vi "find_path.vi"(11 "Array":i16[](array[numeric])) -> (0 "debug array":i32[](array[numeric]), 3 "Array 2":i32[](array[numeric]))   [LabVIEW 2012]
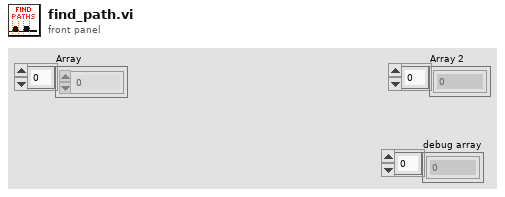
[diagram p1: front panel]
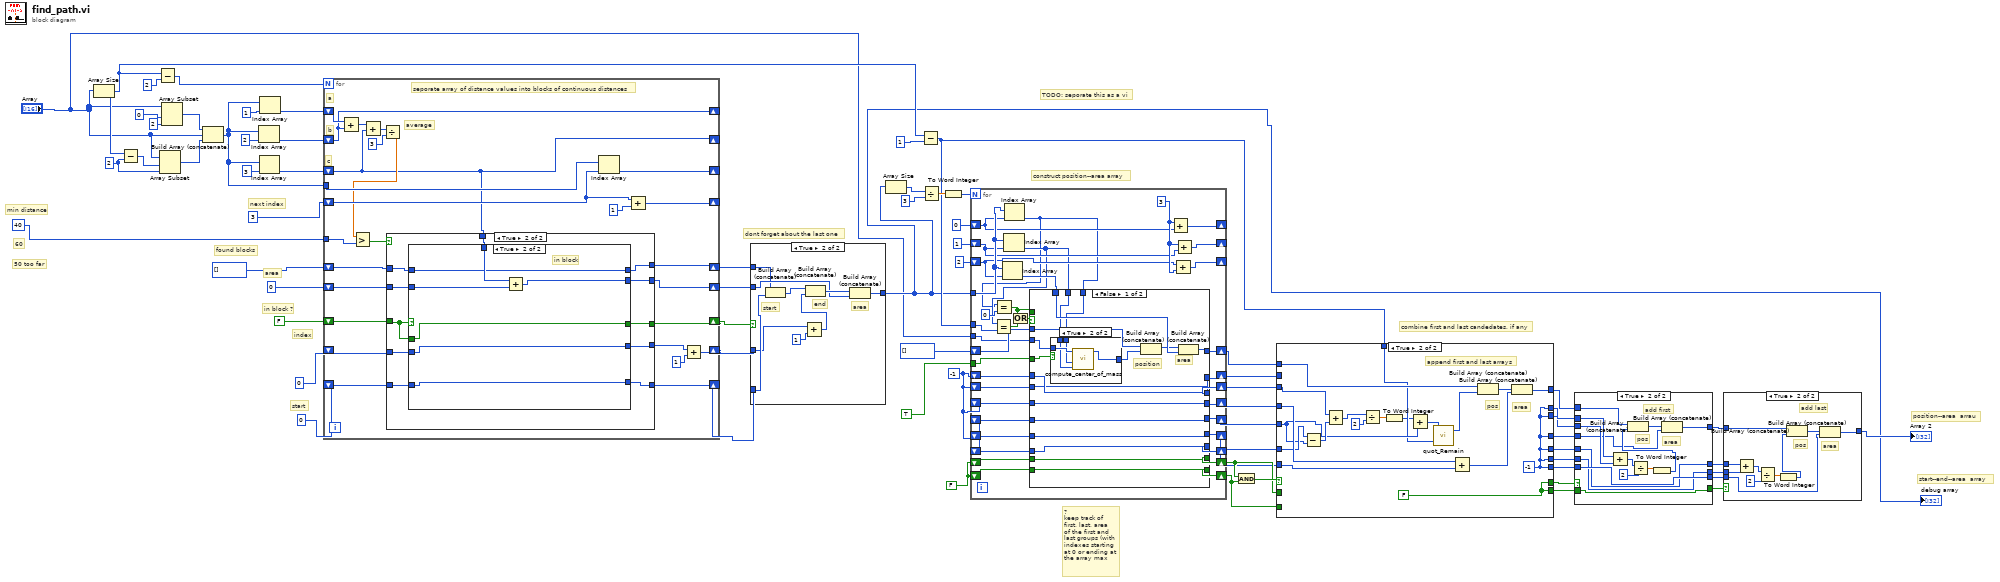
[diagram p0: block diagram]
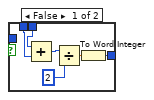
[diagram p5: hidden frame]
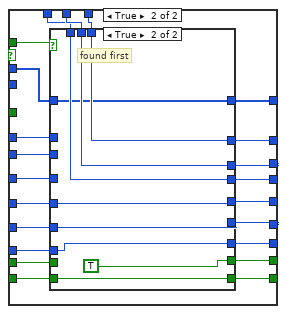
[diagram p6: hidden frame]
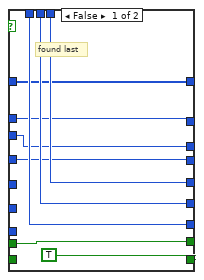
[diagram p7: hidden frame]
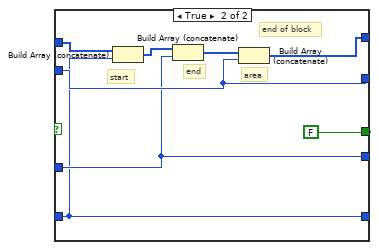
[diagram p10: hidden frame]
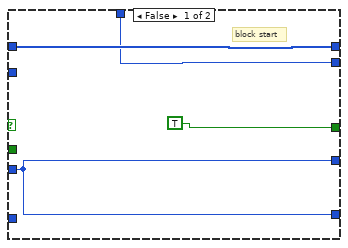
[diagram p11: hidden frame]
diagram:
  w32 = FALSE
  w31 = -1 ("x")
  w64 = 2 ("x")
  # "50 too far"
  # "?\nkeep track of \nfirst, last, area\nof the first and\nlast groups (with\nindexes starting\nat 0 or ending at\nthe array max"
  # "dont forget about the last one"
  # "60"
  # "TODO: seporate this as a vi"
  # "position--area  arrau"
  # "start--end--area  array"
  # "combine first and last candedates, if any"
  # "construct position--area array"
  # "start"
  # "in block ?"
  # "area"
  # "next index"
  # "index"
  # "min distance"
  # "found blocks"
  n1 = Array Size(array="Array") -> (size(s)=w34:i32)
  n2 = Subtract(x=w34, y=w64) -> (x-y=w65:i32)
  n3 = Subtract(x=w34, y=2 ("x")) -> (x-y=w67:i32)
  n4 = Array Subset(array="Array", index=w65, length=w64) -> (w61:i16[])
  n5 = Array Subset(array="Array", index=0 ("x"), length=2 ("x")) -> (w66:i16[])
  n6 = Build Array (concatenate)(w66, "Array", w61) -> (w54:i16[])
  n7 = Index Array(array=w54, index=2 ("x")) -> (element=w56:i16)
  n8 = Index Array(array=w54, index=3 ("x")) -> (element=w55:i16)
  n9 = Index Array(array=w54, index=1 ("x")) -> (element=w57:i16)
  n10 = for {
    N: w67 -> [_]
    shift-right: [w70] -> _
    shift-left: w57 -> [w93]
    shift-right: [w69] -> _
    shift-left: w56 -> [w70]
    shift-right: [w89] -> _
    shift-left: w55 -> [w69]
    tunnel: w54 -> [w90]
    shift-right: [w88] -> _
    shift-left: 3 ("x") -> [w87]
    tunnel: 40 ("x") -> [w83]
    shift-right: [w79] -> w47
    shift-left: FALSE -> [w82]
    shift-right: [w80] -> w44
    shift-left: 0 ("x") -> [w81]
    shift-right: [w76] -> w46
    shift-left: 0 ("x") -> [w78]
    shift-right: [w73] -> w45
    shift-left: 0 ("x") -> [w77]
    shift-right: [w71] -> w43
    shift-left: i16[] [] -> [w75]
    # "seporate array of distance values into blocks of continuous distances"
    # "average"
    # "c"
    # "b"
    # "a"
    n11 = Add(x=w93, y=w70) -> (x+y=w94:i16)
    n12 = Add(x=w94, y=w69) -> (x+y=w92:i16)
    n13 = Divide(x=w92, y=3 ("x")) -> (x/y=w84:dbl)
    n14 = Greater?(x=w84, y=w83) -> (0:w85:bool)
    n15 = case shown="True" w85 {
      tunnel: w82 -> [w104 w125]
      tunnel: w81 -> [w99 w128]
      tunnel: w69 -> [_ w127]
      tunnel: [w98 w126] -> w80
      tunnel: [w103 w124] -> w79
      tunnel: w78 -> [w101 w123]
      tunnel: w77 -> [w100 w122]
      tunnel: [w96 w121] -> w76
      tunnel: w75 -> [w102 w119]
      tunnel: [w97 w120] -> w74
      tunnel: [w95 w118] -> w71
      frame False {
        n16 = case shown="False" w104 {
          selector: w104 -> [w107 _]
          tunnel: [w107 FALSE] -> w103
          tunnel: w102 -> [w109 w116]
          tunnel: w101 -> [w105 w111]
          tunnel: w100 -> [w106 w112]
          tunnel: w99 -> [w108 w113]
          tunnel: [w108 w113] -> w98
          tunnel: [w106 w112] -> w97
          tunnel: [w105 w111] -> w96
          tunnel: [w109 w110] -> w95
          frame False {
          }
          frame True {
            # "area"
            # "end"
            # "start"
            # "end of block"
            n17 = Build Array (concatenate)(w116, w111) -> (w115:i32[])
            n18 = Build Array (concatenate)(w115, w112) -> (w114:i32[])
            n19 = Build Array (concatenate)(w114, w113) -> (w110:i32[])
          }
        }
      }
      frame True {
        n20 = case shown="True" w125 {
          tunnel: w128 -> [_ w139]
          tunnel: w127 -> [w129 w138]
          tunnel: [w129 w137] -> w126
          tunnel: w125 -> [_ w136]
          tunnel: [TRUE w136] -> w124
          tunnel: w123 -> [_ w135]
          tunnel: w122 -> [w131 w134]
          tunnel: [w131 w135] -> w121
          tunnel: [w131 w134] -> w120
          tunnel: w119 -> [w130 w133]
          tunnel: [w130 w133] -> w118
          frame False {
            # "block start"
          }
          frame True {
            # "in block"
            n21 = Add(x=w138, y=w139) -> (x+y=w137:i32)
          }
        }
      }
    }
    n22 = Index Array(array=w90, index=w87) -> (element=w89:i16)
    n23 = Add(x=w87, y=1 ("x")) -> (x+y=w88:i32)
    n24 = Add(x=w74, y=1 ("x")) -> (x+y=w73:i32)
  }
  n25 = case shown="True" w47 {
    tunnel: w46 -> [_ w147]
    tunnel: w45 -> [_ w144]
    tunnel: w44 -> [_ w143]
    tunnel: [w140 w142] -> w3
    tunnel: w43 -> [w140 w141]
    frame False {
    }
    frame True {
      # "area"
      # "end"
      # "start"
      n26 = Build Array (concatenate)(w141, w147) -> (w148:i32[])
      n27 = Add(x=w144, y=1 ("x")) -> (x+y=w145:i32)
      n28 = Build Array (concatenate)(w148, w145) -> (w149:i32[])
      n29 = Build Array (concatenate)(w149, w143) -> (w142:i32[])
    }
  }
  "debug array" <- w3
  n30 = Array Size(array=w3) -> (size(s)=w41:i32)
  n31 = Subtract(x=w34, y=1) -> (x-y=w15:i32)
  n32 = Divide(x=w41, y=3) -> (x/y=w39:dbl)
  n33 = To Word Integer(number=w39) -> (16bit integer=w38:i16)
  n34 = for {
    N: w38 -> [_]
    tunnel: w3 -> [w182]
    shift-right: [w163] -> w18
    shift-left: w31 -> [w175]
    shift-right: [w162] -> w19
    shift-left: w31 -> [w174]
    shift-right: [w161] -> w20
    shift-left: w31 -> [w173]
    shift-right: [w168] -> w21
    shift-left: w31 -> [w172]
    shift-right: [w166] -> w22
    shift-left: w31 -> [w171]
    shift-right: [w164] -> w23
    shift-left: w31 -> [w170]
    shift-right: [w183] -> _
    shift-left: 0 ("x") -> [w169]
    shift-right: [w184] -> _
    shift-left: 1 ("x") -> [w167]
    shift-right: [w185] -> _
    shift-left: 2 ("x") -> [w165]
    tunnel: w15 -> [w176]
    shift-right: [w157] -> w27
    shift-left: w32 -> [w159]
    shift-right: [w158] -> w28
    shift-left: w32 -> [w160]
    shift-right: [w155] -> w17
    shift-left: i16[] [] -> [w156]
    tunnel: "Array" -> [w151]
    tunnel: TRUE -> [w150]
    w181 = 3 ("x")
    n35 = Index Array(array=w182, index=w165) -> (element=w154:i32)
    n36 = Index Array(array=w182, index=w167) -> (element=w153:i32)
    n37 = Equal?(x=w153, y=w176) -> (x = y?=w180:bool)
    n38 = Index Array(array=w182, index=w169) -> (element=w152:i32)
    n39 = Equal?(x=w152, y=0 ("x")) -> (x = y?=w177:bool)
    n40 = Or(x=w177, y=w180) -> (x .or. y?=w179:bool)
    n41 = case shown="False" w179 {
      tunnel: w177 -> [_ w234]
      tunnel: w175 -> [w202 w233]
      tunnel: w174 -> [w201 w232]
      tunnel: w173 -> [w200 w231]
      tunnel: w172 -> [w199 w230]
      tunnel: w171 -> [w198 w229]
      tunnel: w170 -> [w197 w228]
      tunnel: w152 -> [w191 w227]
      tunnel: [w199 w226] -> w168
      tunnel: w153 -> [w192 w225]
      tunnel: [w198 w224] -> w166
      tunnel: w154 -> [w194 w223]
      tunnel: [w197 w222] -> w164
      tunnel: [w202 w221] -> w163
      tunnel: [w201 w220] -> w162
      tunnel: [w200 w219] -> w161
      tunnel: w160 -> [w196 w218]
      tunnel: w159 -> [w195 w217]
      tunnel: [w195 w216] -> w157
      tunnel: [w196 w215] -> w158
      tunnel: w156 -> [w188 w214]
      tunnel: [w193 w213] -> w155
      tunnel: w151 -> [w186 _]
      tunnel: w150 -> [w187 _]
      frame False {
        # "position"
        # "area"
        n42 = case shown="True" w187 {
          tunnel: w192 -> [w208 w209]
          tunnel: w191 -> [w207 w210]
          tunnel: [w206 w212] -> w190
          tunnel: w186 -> [_ w211]
          frame False {
            n43 = Add(x=w207, y=w208) -> (x+y=w205:i32)
            n44 = Divide(x=w205, y=2 ("x")) -> (x/y=w203:dbl)
            n45 = To Word Integer(number=w203) -> (16bit integer=w206:i16)
          }
          frame True {
            n46 = call "compute_center_of_mass.vi"("end"=w209, "start"=w210, "array"=w211) -> ("center of  'mass'"=w212:u16)  [unwired: 8 in]
          }
        }
        n47 = Build Array (concatenate)(w188, w190) -> (w189:i32[])
        n48 = Build Array (concatenate)(w189, w194) -> (w193:i32[])
      }
      frame True {
        n49 = case shown="True" w234 {
          tunnel: w233 -> [w237 _]
          tunnel: w232 -> [w236 _]
          tunnel: w231 -> [w235 _]
          tunnel: w230 -> [_ w249]
          tunnel: w229 -> [_ w248]
          tunnel: w228 -> [_ w247]
          tunnel: w227 -> [w243 w252]
          tunnel: [w243 w249] -> w226
          tunnel: w225 -> [w242 w251]
          tunnel: [w242 w248] -> w224
          tunnel: w223 -> [w241 w250]
          tunnel: [w241 w247] -> w222
          tunnel: [w237 w252] -> w221
          tunnel: [w236 w251] -> w220
          tunnel: [w235 w250] -> w219
          tunnel: w218 -> [w239 _]
          tunnel: w217 -> [_ w246]
          tunnel: [TRUE w246] -> w216
          tunnel: [w239 TRUE] -> w215
          tunnel: w214 -> [w238 w244]
          tunnel: [w238 w244] -> w213
          frame False {
            # "found last"
          }
          frame True {
            # "found first"
          }
        }
      }
    }
    n50 = Add(x=w181, y=w169) -> (x+y=w183:i32)
    n51 = Add(x=w165, y=w181) -> (x+y=w185:i32)
    n52 = Add(x=w181, y=w167) -> (x+y=w184:i32)
  }
  n53 = And(x=w28, y=w27) -> (x .and. y?=w29:bool)
  n54 = case shown="True" w29 {
    tunnel: [w261 w280] -> w26
    tunnel: [w260 w280] -> w25
    tunnel: w28 -> [w261 _]
    tunnel: w27 -> [w260 _]
    tunnel: w23 -> [w258 w275]
    tunnel: w22 -> [w257 w271]
    tunnel: w21 -> [w256 w270]
    tunnel: w20 -> [w255 w276]
    tunnel: w19 -> [w254 w272]
    tunnel: w18 -> [w253 _]
    tunnel: w17 -> [w259 w274]
    tunnel: [w259 w278] -> w16
    tunnel: w15 -> [_ w268]
    tunnel: [w258 w266] -> w9
    tunnel: [w257 w266] -> w10
    tunnel: [w256 w266] -> w11
    tunnel: [w255 w266] -> w12
    tunnel: [w254 w266] -> w13
    tunnel: [w253 w266] -> w14
    frame False {
    }
    frame True {
      w266 = -1 ("x")
      w280 = FALSE
      # "area"
      # "pos"
      # "append first and last arrays"
      n55 = Subtract(x=w271, y=w270) -> (x-y=w273:i32)
      n56 = Add(x=w272, y=w273) -> (x+y=w264:i32)
      n57 = Divide(x=w264, y=2 ("x")) -> (x/y=w263:dbl)
      n58 = To Word Integer(number=w263) -> (16bit integer=w262:i16)
      n59 = Add(x=w262, y=w270) -> (x+y=w269:i32)
      n60 = call <vilib>:"quot_Remain.vi"("y"=w268, "x"=w269) -> ("x-y*floor(x/y)"=w267:i32)  [unwired: 1 out]
      n61 = Add(x=w276, y=w275) -> (x+y=w277:i32)
      n62 = Build Array (concatenate)(w274, w267) -> (w279:i32[])
      n63 = Build Array (concatenate)(w279, w277) -> (w278:i32[])
    }
  }
  n64 = case shown="True" w26 {
    tunnel: w25 -> [w285 w299]
    tunnel: [w285 w299] -> w24
    tunnel: w16 -> [w284 w290]
    tunnel: w14 -> [_ w293]
    tunnel: w13 -> [_ w294]
    tunnel: w12 -> [_ w291]
    tunnel: w11 -> [w281 w286]
    tunnel: w10 -> [w282 w287]
    tunnel: w9 -> [w283 w288]
    tunnel: [w284 w289] -> w8
    tunnel: [w283 w288] -> w5
    tunnel: [w282 w287] -> w6
    tunnel: [w281 w286] -> w7
    frame False {
    }
    frame True {
      # "area"
      # "pos"
      # "add first"
      n65 = Add(x=w293, y=w294) -> (x+y=w296:i32)
      n66 = Divide(x=w296, y=2 ("x")) -> (x/y=w298:dbl)
      n67 = To Word Integer(number=w298) -> (16bit integer=w292:i16)
      n68 = Build Array (concatenate)(w290, w292) -> (w295:i32[])
      n69 = Build Array (concatenate)(w295, w291) -> (w289:i32[])
    }
  }
  n70 = case shown="True" w24 {
    tunnel: w8 -> [w300 w306]
    tunnel: w7 -> [_ w305]
    tunnel: w6 -> [_ w304]
    tunnel: w5 -> [_ w303]
    tunnel: [w300 w301] -> w4
    frame False {
    }
    frame True {
      # "area"
      # "pos"
      # "add last"
      n71 = Add(x=w305, y=w304) -> (x+y=w310:i32)
      n72 = Divide(x=w310, y=2 ("x")) -> (x/y=w308:dbl)
      n73 = To Word Integer(number=w308) -> (16bit integer=w302:i16)
      n74 = Build Array (concatenate)(w306, w302) -> (w307:i32[])
      n75 = Build Array (concatenate)(w307, w303) -> (w301:i32[])
    }
  }
  "Array 2" <- w4
